vi "Line Drawing.vi"(6 "Numeric":i32, 7 "Array in":dbl[](array[numeric]), 9 "Numeric 3":i32, 10 "Numeric 2":dbl, 11 "Numeric 4":dbl) -> (3 "Array out":dbl[](array[numeric]))   [LabVIEW 2017]
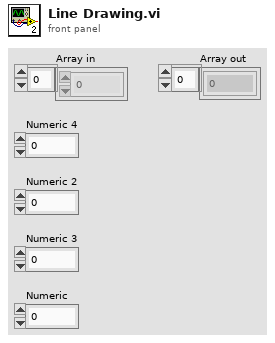
[diagram p1: front panel]
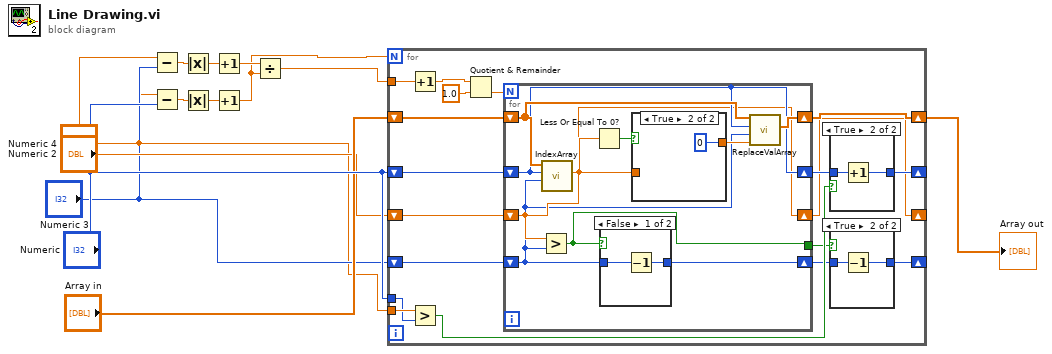
[diagram p0: block diagram]
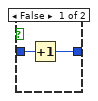
[diagram p2: hidden frame]
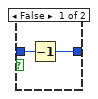
[diagram p3: hidden frame]
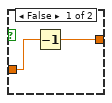
[diagram p4: hidden frame]
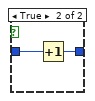
[diagram p5: hidden frame]
diagram:
  n1 = Subtract(x="Numeric 2", y="Numeric 3") -> (x-y=w9:dbl)
  n2 = Subtract(x="Numeric 4", y="Numeric") -> (x-y=w8:dbl)
  n3 = Absolute Value(x=w9) -> (abs(x)=w10:dbl)
  n4 = Absolute Value(x=w8) -> (abs(x)=w7:dbl)
  n5 = Increment(x=w10) -> (x+1=w13:dbl)
  n6 = Increment(x=w7) -> (x+1=w11:dbl)
  n7 = Divide(x=w13, y=w11) -> (x/y=w12:dbl)
  n8 = for {
    N: w11 -> [_]
    tunnel: w12 -> [w19]
    shift-right: [w27] -> _
    shift-left: "Numeric" -> [w29]
    tunnel: "Numeric 4" -> [w31]
    tunnel: "Numeric" -> [w30]
    shift-right: [w24] -> w5
    shift-left: "Array in" -> [w25]
    shift-right: [w14] -> _
    shift-left: "Numeric 3" -> [w23]
    shift-right: [w17] -> _
    shift-left: "Numeric 2" -> [w18]
    n9 = Increment(x=w19) -> (x+1=w20:dbl)
    n10 = Greater?(x=w31, y=w30) -> (0:w26:bool)
    n11 = Quotient & Remainder(x=w20, y=1.0) -> (floor(x/y)=w21:dbl)  [unwired: 1 out]
    n12 = for {
      N: w21 -> [_]
      shift-right: [w49] -> w15
      shift-left: w23 -> [w41]
      shift-right: [w48] -> w24
      shift-left: w25 -> [w47]
      shift-right: [w43] -> w28
      shift-left: w29 -> [w43]
      shift-right: [w42] -> w17
      shift-left: w18 -> [w42]
      tunnel: [w40] -> w16
      n13 = Greater?(x=w42, y=w41) -> (0:w40:bool)
      n14 = call "IndexArray.vi"("y"=w41, "x"=w43, "Array"=w47) -> (2:w44:dbl)  [unwired: 8 in]
      n15 = Less Or Equal To 0?(x=w44) -> (x <= 0?=w46:bool)
      n16 = case shown="False" w40 {
        tunnel: w41 -> [w53 w56]
        tunnel: [w54 w55] -> w49
        frame False {
          n17 = Decrement(x=w53) -> (x-1=w54:i32)
        }
        frame True {
          n18 = Increment(x=w56) -> (x+1=w55:i32)
        }
      }
      n19 = case shown="True" w46 {
        tunnel: [w51 0] -> w45
        tunnel: w44 -> [w50 _]
        frame False {
          n20 = Decrement(x=w50) -> (x-1=w51:dbl)
        }
        frame True {
        }
      }
      n21 = call "ReplaceValArray.vi"("Value"=w45, "y"=w41, "x"=w43, "Array"=w47) -> ("output array"=w48:dbl[])  [unwired: 7 in]
    }
    n22 = case shown="True" w26 {
      tunnel: w28 -> [w36 w39]
      tunnel: [w37 w38] -> w27
      frame False {
        n23 = Decrement(x=w36) -> (x-1=w37:i32)
      }
      frame True {
        n24 = Increment(x=w39) -> (x+1=w38:i32)
      }
    }
    n25 = case shown="True" w16 {
      tunnel: w15 -> [w33 w34]
      tunnel: [w32 w35] -> w14
      frame False {
        n26 = Increment(x=w33) -> (x+1=w32:i32)
      }
      frame True {
        n27 = Decrement(x=w34) -> (x-1=w35:i32)
      }
    }
  }
  "Array out" <- w5
